vi "Set Key Value (Control Value).vi"(5 "Key name":string, 6 "Control reference":refnum<vi>, 7 "Section name":string, 8 "error in (no error)":errorcluster, 9 "Create key? [T]":bool=TRUE, 10 "Create section? [T]":bool=TRUE, 11 "Carya Config in":refnum<class "Carya Config.lvclass">) -> (0 "error out":errorcluster, 1 "Created key?":bool, 2 "Created session?":bool, 3 "Carya Config out":refnum<class "Carya Config.lvclass">, 4 "Value written?":bool)   [LabVIEW 2013, in "Carya Config.lvclass"]
doc: "Copyright 2018, Carya Automatisering, Wiebe Walstra."
uses:
  Carya Config.lvclass
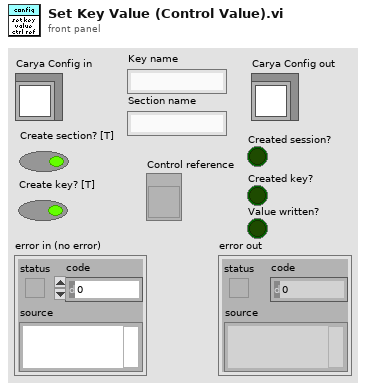
[diagram p1: front panel]
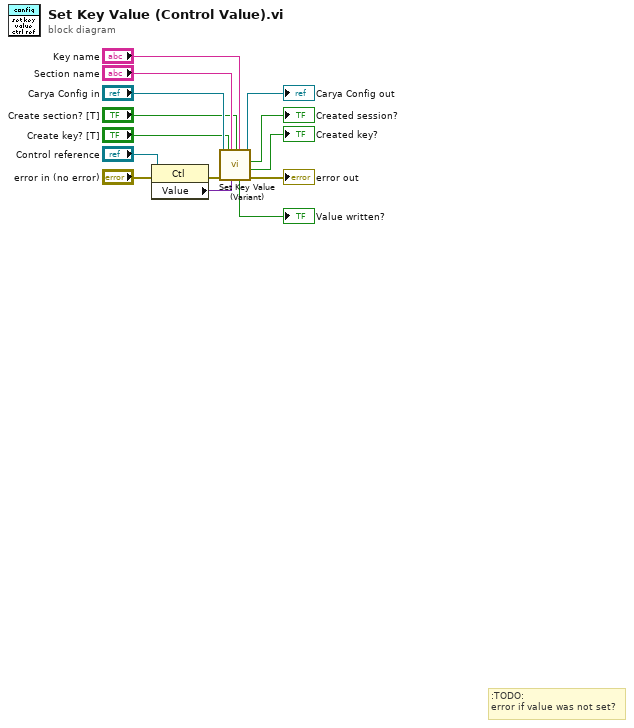
[diagram p0: block diagram]
diagram:
  # ":TODO:\nerror if value was not set?"
  n1 = property class="Ctl"(reference="Control reference", error in="error in (no error)") -> (error out=w2:errorcluster, "Value"=w4:variant)  [unwired: 1 out]
  n2 = call "Set Key Value (Variant).vi"("Key name"="Key name", "Key value"=w4, "Section name"="Section name", "error in (no error)"=w2, "Create key? [T]"="Create key? [T]", "Create section? [T]"="Create section? [T]", "Carya Config in"="Carya Config in") -> ("error out"=→"error out":errorcluster, "Created key?"=→"Created key?":bool, "Created session?"=→"Created session?":bool, "Carya Config out"=→"Carya Config out":refnum<class "Carya Config.lvclass">, "Value written?"=→"Value written?":bool)
